vi "Radau5_Manager.vi"(9 "Jac Variant":variant, 10 "Jac Refnum":refnum<vi>, 11 "Simulation Data In":T1 {"Absolute tolerance" format="%.1e"; "Relative tolerance" format="%.1e"; "Output of T" format="%.1e"; "proposed step size" format="%.1e"; "min step size" format="%.1e"; "max step size" format="%.1e"; "final time" format="%.1e"; "step size" format="%.1e"; "initial time" format="%.1e"}) -> (2 "step complete?":bool, 3 "Simulation Data Out":T1 {"Absolute tolerance" format="%.1e"; "Relative tolerance" format="%.1e"; "Output of T" format="%.1e"; "proposed step size" format="%.1e"; "min step size" format="%.1e"; "max step size" format="%.1e"; "final time" format="%.1e"; "step size" format="%.1e"; "initial time" format="%.1e"})   [LabVIEW 2020, in "NI_DAE.lvlib"]
doc: "<B>DAE manager</B> is DAE solver core, where different solver algorithms are."
uses:
  <vilib>/gmath/NI_DAE.lvlib
  <vilib>/gmath/dae.llb/Radau5_Simulation Data.ctl
  <vilib>/gmath/dae.llb/Radau5_Diag Eval Stage.ctl
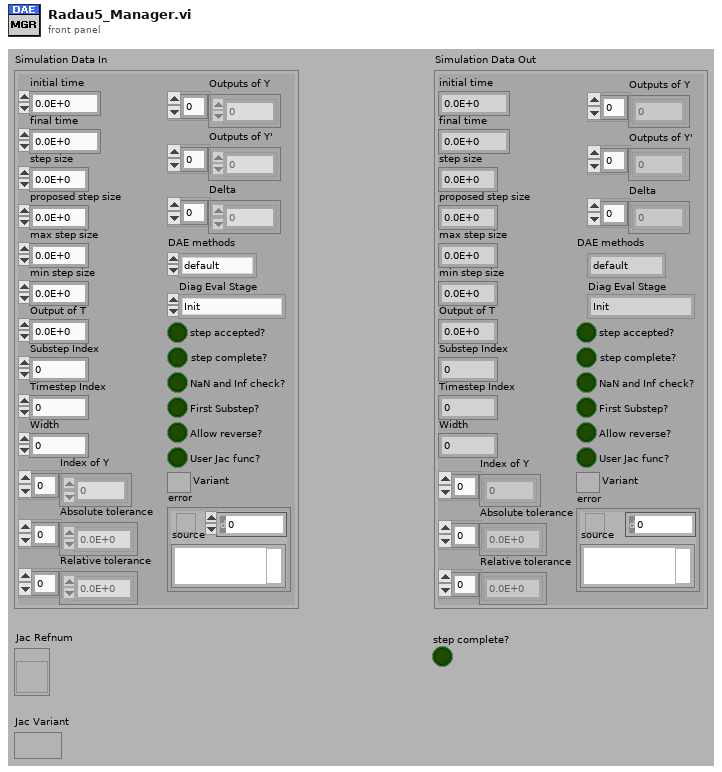
[diagram p1: front panel]
types:
  T1 = typedef "NI_DAE.lvlib/Radau5_Simulation Data.ctl" = cluster{"initial time":dbl, "final time":dbl, "step size":dbl, "proposed step size":dbl, "max step size":dbl, "min step size":dbl, "Output of T":dbl, "Substep Index":i32, "Timestep Index":i32, "Width":i32, "Absolute tolerance":dbl[], "Relative tolerance":dbl[], "Outputs of Y":dbl[], "Outputs of Y'":dbl[], "Delta":dbl[], "DAE methods":enum16{"default", "Radau IIA"}, "Diag Eval Stage":T2, "step accepted?":bool, "step complete?":bool, "NaN and Inf check?":bool, "First Substep?":bool, "Allow reverse?":bool, "error":errorcluster, "User Jac func?":bool, "Variant":variant, "Index of Y":i8[]}
  T2 = typedef "NI_DAE.lvlib/Radau5_Diag Eval Stage.ctl" = enum16{"Init", "Running", "Final", "End"}
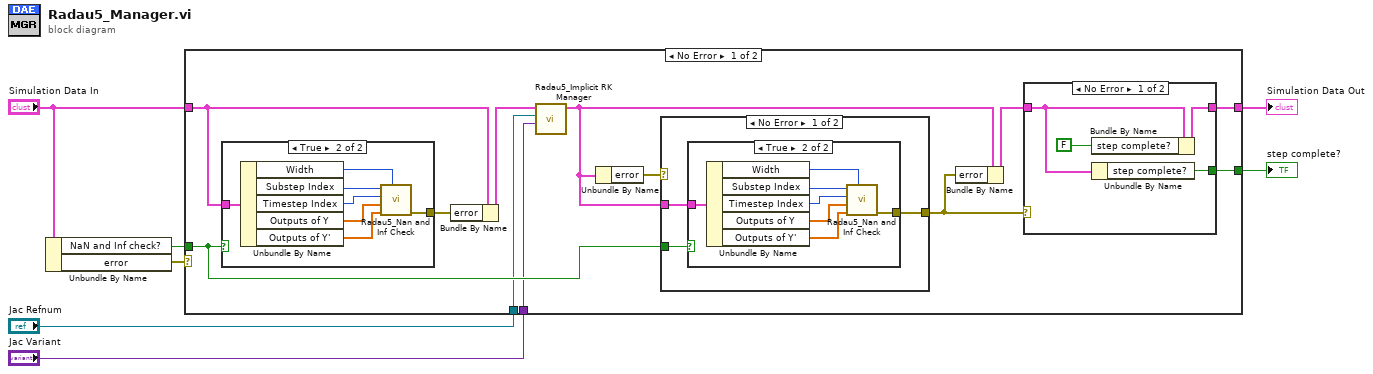
[diagram p0: block diagram]
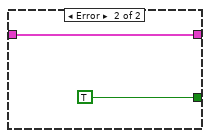
[diagram p2: hidden frame]
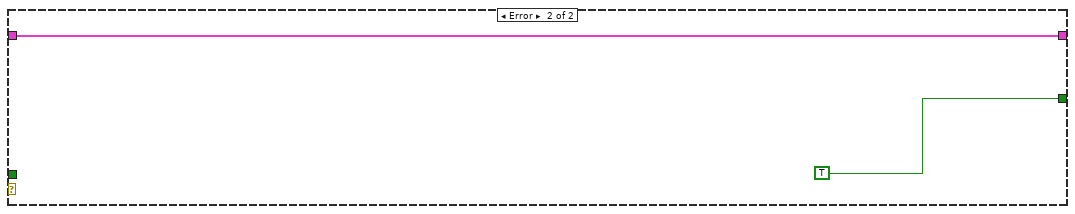
[diagram p6: hidden frame]
diagram:
  n1 = Unbundle By Name("Simulation Data In") -> ("NaN and Inf check?"=w7:bool, "error"=w5:errorcluster)
  n2 = case shown="No Error" w5 {
    tunnel: w7 -> [w16 _]
    tunnel: "Simulation Data In" -> [w18 w44]
    tunnel: [w11 w44] -> w4
    tunnel: [w10 TRUE ("step complete?")] -> w3
    tunnel: "Jac Refnum" -> [w9 _]
    tunnel: "Jac Variant" -> [w8 _]
    frame No Error {
      n3 = case shown="True" w16 {
        tunnel: w18 -> [_ w43]
        tunnel: [_ w38] -> w19
        frame False {
        }
        frame True {
          n4 = Unbundle By Name(w43) -> ("Width"=w37:i32, "Substep Index"=w42:i32, "Timestep Index"=w41:i32, "Outputs of Y"=w40:dbl[], "Outputs of Y'"=w39:dbl[])
          n5 = call <vilib>:"Radau5_Nan and Inf Check.vi"("Width"=w37, "Input Array Y'"=w39, "Input Array Y"=w40, "Time Index"=w41, "SubIndex"=w42) -> ("error out"=w38:errorcluster)  [unwired: 6 in]
        }
      }
      n6 = Bundle By Name(cluster=w18, "error"=w19) -> (w17:T1)
      n7 = call <vilib>:"Radau5_Implicit RK Manager.vi"("Jac Variant"=w8, "Jac Refnum"=w9, "Simulation Data In"=w17) -> ("Simulation Data Out"=w15:T1)  [unwired: 8 in]
      n8 = Unbundle By Name(w15) -> ("error"=w14:errorcluster)
      n9 = case shown="No Error" w14 {
        selector: w14 -> [_ w36]
        tunnel: w16 -> [w26 _]
        tunnel: [w27 w36] -> w13
        tunnel: w15 -> [w28 _]
        frame No Error {
          n10 = case shown="True" w26 {
            tunnel: w28 -> [_ w35]
            tunnel: [_ w30] -> w27
            frame False {
            }
            frame True {
              n11 = Unbundle By Name(w35) -> ("Width"=w29:i32, "Substep Index"=w34:i32, "Timestep Index"=w33:i32, "Outputs of Y"=w32:dbl[], "Outputs of Y'"=w31:dbl[])
              n12 = call <vilib>:"Radau5_Nan and Inf Check.vi"("Width"=w29, "Input Array Y'"=w31, "Input Array Y"=w32, "Time Index"=w33, "SubIndex"=w34) -> ("error out"=w30:errorcluster)  [unwired: 6 in]
            }
          }
        }
        frame Error {
        }
      }
      n13 = Bundle By Name(cluster=w15, "error"=w13) -> (w12:T1)
      n14 = case shown="No Error" w13 {
        tunnel: [w20 w25] -> w11
        tunnel: w12 -> [w22 w25]
        tunnel: [w23 TRUE ("step complete?")] -> w10
        frame No Error {
          n15 = Bundle By Name(cluster=w22, "step complete?"=FALSE) -> (w20:T1)
          n16 = Unbundle By Name(w22) -> ("step complete?"=w23:bool)
        }
        frame Error {
        }
      }
    }
    frame Error {
    }
  }
  "Simulation Data Out" <- w4
  "step complete?" <- w3
